vi "Moves Forward.vi"(7 "yaw setpoint":dbl format="%#_13g", 8 "error in (no error)":errorcluster, 9 "Speed":dbl, 10 "forwardDistance":dbl, 11 "PID gains":T1) -> (0 "error out":errorcluster, 2 "EncoderDevRef":T2, 3 "EncoderDevRef 2":T2)   [LabVIEW 2017]
uses:
  <vilib>/Rock Robotics/WPI/Encoder/WPI_EncoderDevRef.ctl
  <vilib>/Rock Robotics/SystemInterfaces/Encoder/FPGA_EncoderIdx.ctl
  <vilib>/Rock Robotics/SystemInterfaces/Counter/FPGA_CounterCtrSystemIndex.ctl
  <vilib>/Rock Robotics/WPI/Encoder/WPI_EncoderType.ctl
  Documents/LabVIEW Data/Retro 2018/Robot Global Data.vi
  <vilib>/Rock Robotics/Network Tables/NT Write Number.vi
  <vilib>/addons/control/pid/pid.llb/PID (DBL).vi
  <vilib>/addons/control/pid/NI_PID_pid.lvlib
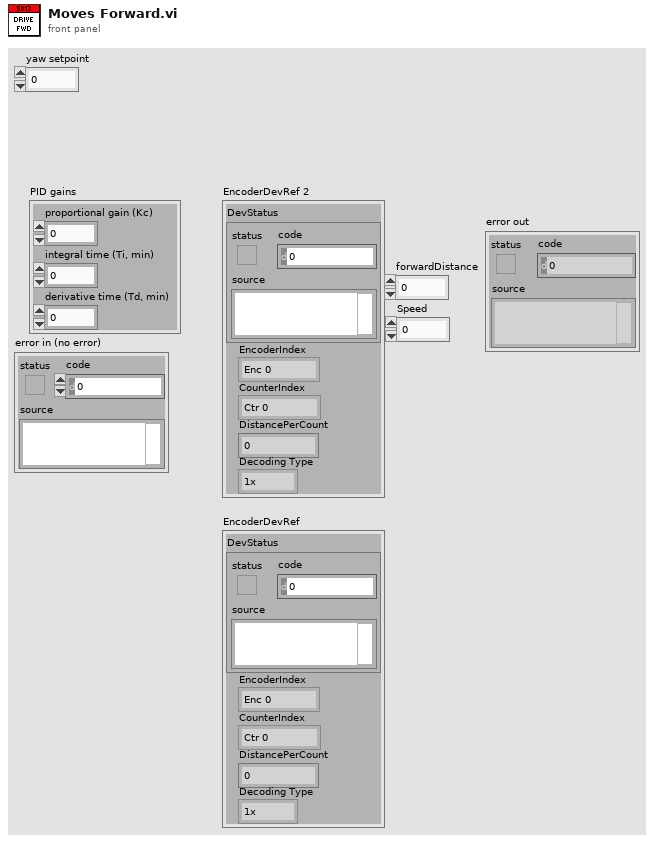
[diagram p1: front panel]
types:
  T1 = cluster{"proportional gain (Kc)":dbl, "integral time (Ti, min)":dbl, "derivative time (Td, min)":dbl}
  T2 = typedef "WPI_EncoderDevRef.ctl" = cluster{"DevStatus":errorcluster, "EncoderIndex":T3, "CounterIndex":T4, "DistancePerCount":dbl, "Decoding Type":T5}
  T3 = typedef "FPGA_EncoderIdx.ctl" = enum8{"Enc 0", "Enc 1", "Enc 2", "Enc 3", "Enc 4", "Enc 5", "Enc 6", "Enc 7", "Invalid"}
  T4 = typedef "FPGA_CounterCtrSystemIndex.ctl" = enum8{"Ctr 0", "Ctr 1", "Ctr 2", "Ctr 3", "Ctr 4", "Ctr 5", "Ctr 6", "Ctr 7", "Invalid"}
  T5 = typedef "WPI_EncoderType.ctl" = enum16{"1x", "2x", "4x"}
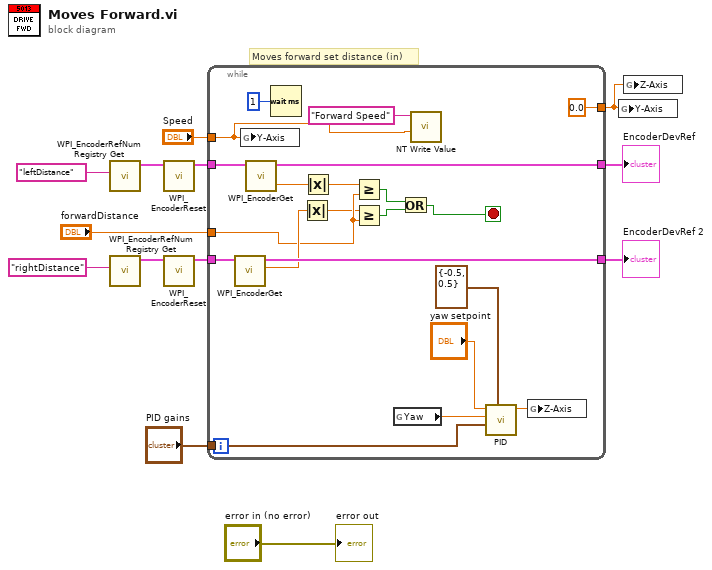
[diagram p0: block diagram]
diagram:
  # "Moves forward set distance (in)"
  n1 = call <vilib>:"WPI_EncoderRefNum Registry Get.vi"("refnum name"="leftDistance") -> ("EncoderDevRef"=w3:T2)  [unwired: 9 in, 1 out]
  n2 = call <vilib>:"WPI_EncoderRefNum Registry Get.vi"("refnum name"="rightDistance") -> ("EncoderDevRef"=w5:T2)  [unwired: 9 in, 1 out]
  n3 = call <vilib>:"WPI_EncoderReset.vi"("EncoderDevRef"=w3) -> ("EncoderDevRef"=w2:T2)  [unwired: 9 in, 1 out]
  n4 = call <vilib>:"WPI_EncoderReset.vi"("EncoderDevRef"=w5) -> ("EncoderDevRef"=w4:T2)  [unwired: 9 in, 1 out]
  n5 = while {
    tunnel: w2 -> [w26]
    tunnel: w4 -> [w27]
    tunnel: [w30] -> w12
    tunnel: [w34] -> w13
    tunnel: "PID gains" -> [w32]
    tunnel: "forwardDistance" -> [w21]
    tunnel: "Speed" -> [w14]
    tunnel: [0.0 ("setpoint")] -> w1
    stop <- w24 stop-if-true
    n6 = call <vilib>:"WPI_EncoderGet.vi"("EncoderDevRef"=w27) -> ("Distance"=w22:dbl, "EncoderDevRef"=w30:T2)  [unwired: 5 in, 4 out]
    n7 = global write "Robot Global Data.vi" "Y-Axis"(w14) -> ()
    n8 = call <vilib>:"WPI_EncoderGet.vi"("EncoderDevRef"=w26) -> ("Distance"=w23:dbl, "EncoderDevRef"=w34:T2)  [unwired: 5 in, 4 out]
    n9 = Wait (ms)(milliseconds to wait=u32 1) -> ()  [unwired: 1 out]
    n10 = Absolute Value(x=w22) -> (abs(x)=w16:dbl)
    n11 = Absolute Value(x=w23) -> (abs(x)=w18:dbl)
    n12 = Greater Or Equal?(x=w18, y=w21) -> (x >= y?=w20:bool)
    n13 = Greater Or Equal?(x=w16, y=w21) -> (x >= y?=w19:bool)
    n14 = global read "Robot Global Data.vi" "Yaw"() -> (w17:dbl)
    n15 = Or(x=w20, y=w19) -> (x .or. y?=w24:bool)
    n16 = call-poly <vilib>:"NT Write Value.vi"("Numeric"=w14, "Name"="Forward Speed") -> ()  [unwired: 9 in, 1 out]
    n17 = call-poly <vilib>:"PID.vi"("output range"=cluster{"output high":dbl, "output low":dbl} {"output high"=-0.5, "output low"=0.5}, "PID gains"=w32, "process variable"=w17, "setpoint"="yaw setpoint") -> ("output"=w31:dbl)  [unwired: 6 in, 1 out]
    n18 = global write "Robot Global Data.vi" "Z-Axis"(w31) -> ()
  }
  "EncoderDevRef" <- w13
  "EncoderDevRef 2" <- w12
  n19 = global write "Robot Global Data.vi" "Y-Axis"(w1) -> ()
  n20 = global write "Robot Global Data.vi" "Z-Axis"(w1) -> ()
  "error out" <- "error in (no error)"
